vi "color deco as temp indicator.vi"(0 "vi path":path, 2 "default BG Color":u32(colorbox)=10842245, 7 "deco index to alter":i32, 11 "Color status":T2 caption="Temperature control status", 13 "exec.T mode":T1, 14 "dynamic color":bool) -> (4 "Num of decos":i32, 15 "FG Color":u32(colorbox))   [LabVIEW 2019]
doc: "This is a Bug C(T) subVI.\n\nThis subVI modifies the color of a decoration in the calling VI according to a temperature color scheme.\n\nPaul K Dixon\nP3600\nCSUSB Physics"
uses:
  typedefs/temp control status.ctl
  typedefs/temp mode enum.ctl
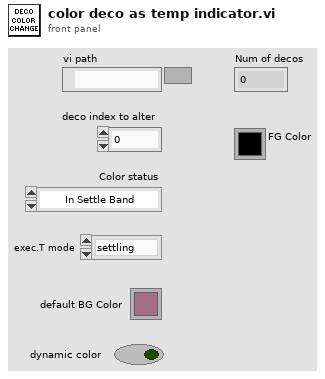
[diagram p1: front panel]
types:
  T1 = typedef "temp mode enum.ctl" = enum16{"settling", "measuring", "holding", "Exit"}
  T2 = typedef "temp control status.ctl" = enum16{"In Settle Band", "In Control Band", "Below Control Band", "Above Control Band"}
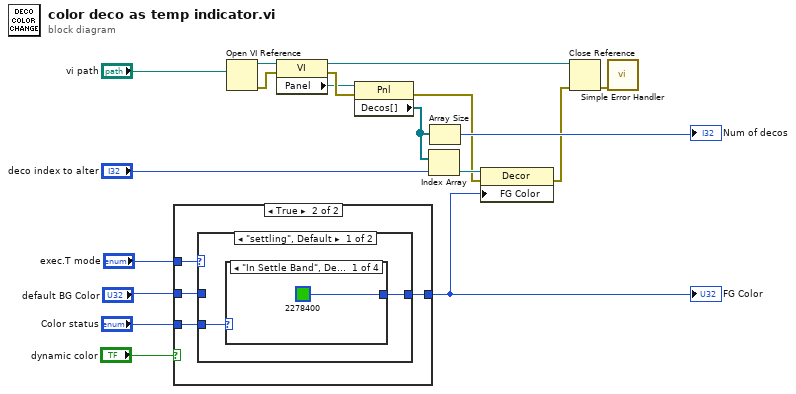
[diagram p0: block diagram]
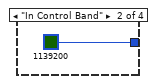
[diagram p3: hidden frame]
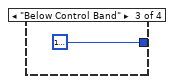
[diagram p4: hidden frame]
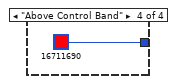
[diagram p5: hidden frame]
diagram:
  n1 = case shown="True" "dynamic color" {
    tunnel: "Color status" -> [_ w23]
    tunnel: [w19 w22] -> w14
    tunnel: "exec.T mode" -> [_ w21]
    tunnel: "default BG Color" -> [w19 w20]
    frame False {
    }
    frame True {
      n2 = case shown="\"settling\", Default" w21 {
        tunnel: w23 -> [w25 _]
        tunnel: [w24 w30] -> w22
        tunnel: w20 -> [_ w30]
        frame "settling", Default {
          n3 = case shown="\"In Settle Band\", Default" w25 {
            tunnel: [u32 2278400 ("BG Color") u32 1139200 ("BG Color") u32 16777224 ("BG Color") u32 16711690 ("BG Color")] -> w24
            frame "In Settle Band", Default {
            }
            frame "In Control Band" {
            }
            frame "Below Control Band" {
            }
            frame "Above Control Band" {
            }
          }
        }
        frame "Exit" {
        }
      }
    }
  }
  "FG Color" <- w14
  n4 = Open VI Reference(vi path="vi path") -> (vi reference=w5:refnum<vi>, error out=w7:errorcluster)  [unwired: 5 in]
  n5 = property class="VI"(reference=w5, error in=w7) -> (reference out=w6:refnum<vi>, error out=w10:errorcluster, "Panel"=w9:refnum<vi>)
  n6 = property class="Pnl"(reference=w9, error in=w10) -> (error out=w11:errorcluster, "Decos[]"=w15:refnum<vi>[])  [unwired: 1 out]
  n7 = Index Array(array=w15, index="deco index to alter") -> (element=w13:refnum<vi>)
  n8 = Array Size(array=w15) -> (size(s)=→"Num of decos":i32)
  n9 = property class="Decor"(reference=w13, error in=w11, "FG Color"=w14) -> (error out=w12:errorcluster)  [unwired: 1 out]
  n10 = Close Reference(reference=w6, error in (no error)=w12) -> (error out=w8:errorcluster)
  n11 = call <vilib>:"Simple Error Handler.vi"("error in (no error)"=w8) -> ()  [unwired: 4 in, 5 out]
